vi "MGI Read Key (i32[]).vi"(7 "Section":string, 8 "error in (no error)":errorcluster, 9 "Default Value[]":i32[](array[numeric]), 10 "Key":string, 11 "Refnum":T1) -> (0 "error out":errorcluster, 1 "Value[]":i32[](array[numeric]), 2 "Found?":bool, 3 "Refnum":T1)   [LabVIEW 2016]
doc: "Read a 1D I32 array key (actually a section) written by the matching Write VI.\n\nAuthored by David A. Moore\nsupport@mooregoodideas.com\nwww.mooregoodideas.com\n\nCopyright (c) 2010, Moore Good Ideas, Inc.\n\nAll rights reserved.\n\nRedistribution and use in source and binary forms, with or without modification, are permitted provided that the following conditions are met:\n\n * Redistributions of source code must retain the above copyright notice, this list of conditions and the following disclaimer.\n * Redistributions in binary form must reproduce the above copyright notice, this list of conditions and the following disclaimer in the documentation and/or other materials provided with the distribution.\n * Neither the name of Moore Good Ideas, Inc. nor the names of its contributors may be used to endorse or promote products derived from this software without specific prior written permission.\n\nTHIS SOFTWARE IS PROVIDED BY THE COPYRIGHT HOLDERS AND CONTRIBUTORS \"AS IS\" AND ANY EXPRESS OR IMPLIED WARRANTIES, INCLUDING, BUT NOT LIMITED TO, THE IMPLIED WARRANTIES OF MERCHANTABILITY AND FITNESS FOR A PARTICULAR PURPOSE ARE DISCLAIMED. IN NO EVENT SHALL THE COPYRIGHT OWNER OR CONTRIBUTORS BE LIABLE FOR ANY DIRECT, INDIRECT, INCIDENTAL, SPECIAL, EXEMPLARY, OR CONSEQUENTIAL DAMAGES (INCLUDING, BUT NOT LIMITED TO, PROCUREMENT OF SUBSTITUTE GOODS OR SERVICES; LOSS OF USE, DATA, OR PROFITS; OR BUSINESS INTERRUPTION) HOWEVER CAUSED AND ON ANY THEORY OF LIABILITY, WHETHER IN CONTRACT, STRICT LIABILITY, OR TORT (INCLUDING NEGLIGENCE OR OTHERWISE) ARISING IN ANY WAY OUT OF THE USE OF THIS SOFTWARE, EVEN IF ADVISED OF THE POSSIBILITY OF SUCH DAMAGE."
uses:
  <vilib>/Utility/config.llb/Config Data RefNum.ctl
  <vilib>/Utility/config.llb/Read Key (I32).vi
  <vilib>/Utility/config.llb/NI_LVConfig.lvlib
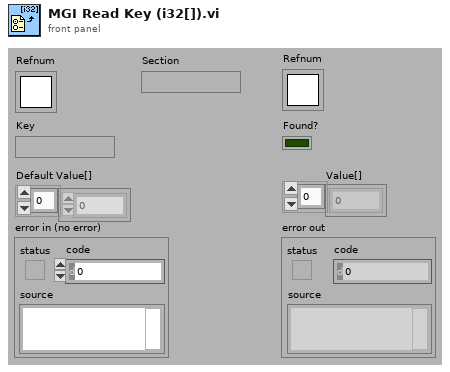
[diagram p1: front panel]
types:
  T1 = typedef "NI_LVConfig.lvlib/Config Data RefNum.ctl" = refnum<k1>
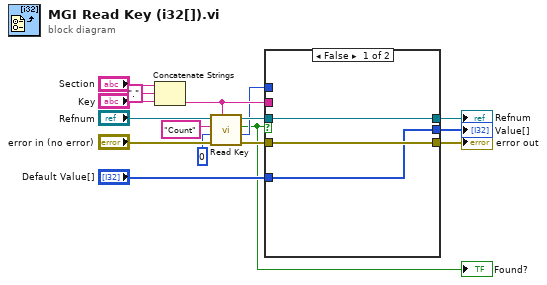
[diagram p0: block diagram]
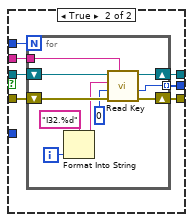
[diagram p2: hidden frame]
diagram:
  n1 = Concatenate Strings("Section", "." ("Substring"), "Key") -> (w8:string)
  n2 = call-poly <vilib>:"Read Key.vi"("section"=w8, "error in (no error)"="error in (no error)", "default value"=0, "key"="Count", "refnum"="Refnum") -> ("error out"=w15:errorcluster, "value"=w4:i32, "found?"=w1:bool, "refnum out"=w14:T1)  [unwired: 3 in]
  "Found?" <- w1
  n3 = case shown="False" w1 {
    tunnel: w15 -> [w18 w26]
    tunnel: w14 -> [w19 w25]
    tunnel: [w18 w24] -> w13
    tunnel: [w19 w23] -> w12
    tunnel: w8 -> [_ w22]
    tunnel: w4 -> [_ w21]
    tunnel: [w17 w20] -> w3
    tunnel: "Default Value[]" -> [w17 _]
    frame False {
    }
    frame True {
      n4 = for {
        N: w21 -> [_]
        shift-right: [w33] -> w24
        shift-left: w26 -> [w36]
        shift-right: [w32] -> w23
        shift-left: w25 -> [w35]
        tunnel: w22 -> [w34]
        tunnel: [w27] -> w20 mode=indexing
        i -> [w31]
        n5 = Format Into String(format string="I32.%d" ("Format String"), w31) -> (resulting string=w30:string)  [unwired: 2 in, 1 out]
        n6 = call-poly <vilib>:"Read Key.vi"("section"=w34, "error in (no error)"=w36, "default value"=0, "key"=w30, "refnum"=w35) -> ("error out"=w33:errorcluster, "value"=w27:i32, "refnum out"=w32:T1)  [unwired: 3 in, 1 out]
      }
    }
  }
  "Value[]" <- w3
  "error out" <- w13
  "Refnum" <- w12
